vi "ReadAccelerometer.vi"(11 "Accelerometer Queue":refnum<queue>) -> (0 "error out":errorcluster)   [LabVIEW 2013]
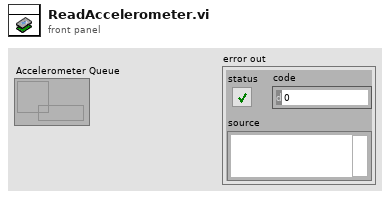
[diagram p1: front panel]
types:
  T1 = cluster{"X-Axis Acceleration":dbl, "Y-Axis Acceleration":dbl, "Z-Axis Acceleration":dbl}
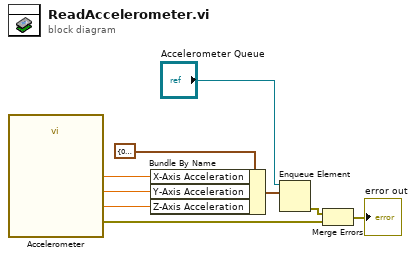
[diagram p0: block diagram]
diagram:
  n1 = call "Accelerometer"() -> ("X-Axis"=w7:dbl, "Y-Axis"=w6:dbl, "Z-Axis"=w5:dbl, "error out"=w3:errorcluster)  [unwired: 24 in]
  n2 = Bundle By Name(cluster=T1 {"X-Axis Acceleration"=0.0, "Y-Axis Acceleration"=0.0, "Z-Axis Acceleration"=0.0} ("output cluster"), "X-Axis Acceleration"=w7, "Y-Axis Acceleration"=w6, "Z-Axis Acceleration"=w5) -> (w4:T1)
  n3 = Enqueue Element(queue="Accelerometer Queue", element=w4) -> (error out=w2:errorcluster)  [unwired: 2 in, 2 out]
  n4 = Merge Errors(w2, w3) -> (→"error out":errorcluster)
